vi "Switch Counter Signal.vi"(4 "Valid Signal Name":string, 5 "Counter Valid GUID":string, 6 "Counter Valid Name":string, 7 "Incoming Frame GUID":string, 8 "error in (no error)":errorcluster, 9 "Signal Page GUID":string, 10 "Counter Value GUID":string, 11 "Node Ptr":T1 format="%.0x") -> (0 "error out":errorcluster)   [LabVIEW 2015, in "Protection and Counter Support System Explorer.lvlib"]
uses:
  Protection and Counter Support System Explorer.lvlib
  <vilib>/NI Veristand/Custom Device API/Custom Device Item Ref.ctl
  <vilib>/NI Veristand/Custom Device API/Custom Device Channel Type.ctl
  <vilib>/NI Veristand/Custom Device API/Custom Device Channel.ctl
  Shared/Properties Lookup.vi
  <vilib>/NI Veristand/Custom Device API/Set Item Property (String).vi
  <vilib>/NI VeriStand/Custom Device API/Custom Device API.lvlib
  <vilib>/NI VeriStand/Custom Device Tools/Custom Device Utility Library/Custom Device Utility Library.lvlib
  Shared/Protection and Counter Support Shared.lvlib
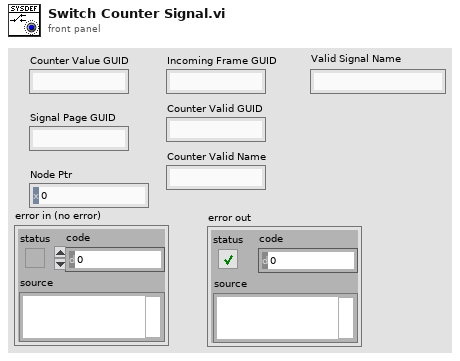
[diagram p1: front panel]
types:
  T1 = typedef "Custom Device API.lvlib/Custom Device Item Ref.ctl" = u64
  T2 = typedef "Custom Device API.lvlib/Custom Device Channel Type.ctl" = enum16{"Input", "Output"}
  T3 = typedef "Custom Device API.lvlib/Custom Device Channel.ctl" = cluster{"Type":T2, "Units":string, "Default Value":dbl, "Faultable":bool, "Scalable":bool}
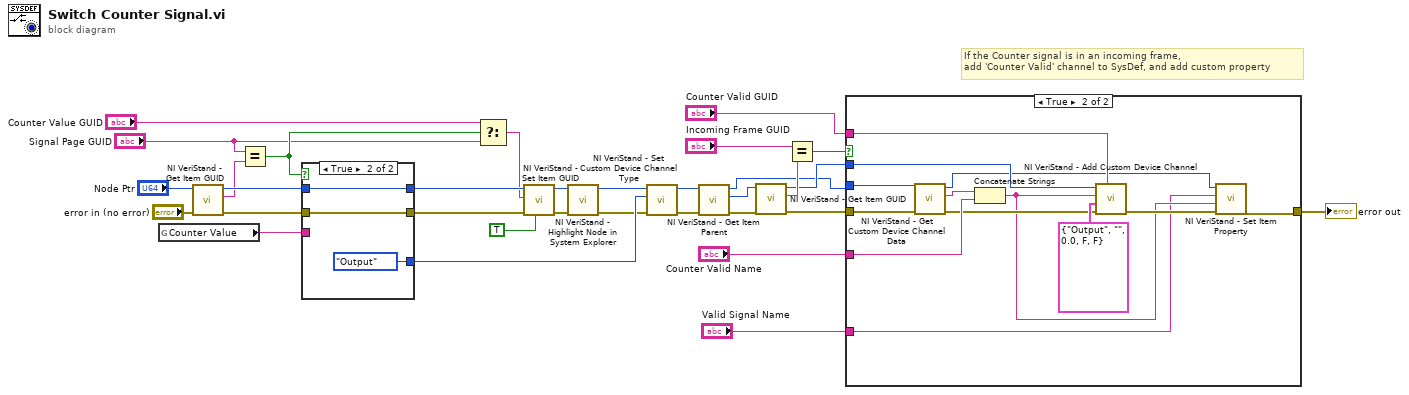
[diagram p0: block diagram]
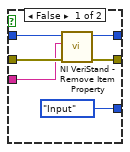
[diagram p3: hidden frame]
diagram:
  # "If the Counter signal is in an incoming frame,\nadd 'Counter Valid' channel to SysDef, and add custom property"
  n1 = global read "Properties Lookup.vi" "Counter Value"() -> (w29:string)
  n2 = call <vilib>:"NI VeriStand - Get Item GUID.vi"("error in (no error)"="error in (no error)", "Item Ref in"="Node Ptr") -> ("error out"=w24:errorcluster, "GUID"=w17:string, "Item Ref out"=w26:T1)  [unwired: 7 in]
  n3 = Equal?(x="Signal Page GUID", y=w17) -> (x = y?=w28:bool)
  n4 = case shown="True" w28 {
    tunnel: w24 -> [w38 w40]
    tunnel: [w37 w40] -> w25
    tunnel: w26 -> [w36 w41]
    tunnel: [w35 w41] -> w27
    tunnel: w29 -> [w34 _]
    tunnel: [Custom_Device_Channel_Type."Input" ("Type") Custom_Device_Channel_Type."Output" ("Type")] -> w32
    frame False {
      n5 = call <vilib>:"NI VeriStand - Remove Item Property.vi"("error in (no error)"=w38, "Property Name"=w34, "Item Ref in"=w36) -> ("error out"=w37:errorcluster, "Item Ref out"=w35:T1)  [unwired: 6 in, 1 out]
    }
    frame True {
    }
  }
  n6 = Select(t="Counter Value GUID", s=w28, f="Signal Page GUID") -> (s? t:f=w19:string)
  n7 = call <vilib>:"NI VeriStand - Set Item GUID.vi"("Refresh System Explorer Tree? (F)"=TRUE, "error in (no error)"=w25, "GUID"=w19, "Item Ref in"=w27) -> ("error out"=w22:errorcluster, "Item Ref out"=w23:T1)  [unwired: 6 in]
  n8 = call <vilib>:"NI VeriStand - Highlight Node in System Explorer.vi"("error in (no error)"=w22, "Item Ref in"=w23) -> ("error out"=w30:errorcluster, "Node Ptr dup"=w31:T1)  [unwired: 8 in]
  n9 = call <vilib>:"NI VeriStand - Set Custom Device Channel Type.vi"("error in (no error)"=w30, "Type"=w32, "Channel Ref in"=w31) -> ("error out"=w14:errorcluster, "Channel Ref out"=w13:T1)  [unwired: 7 in]
  n10 = call <vilib>:"NI VeriStand - Get Item Parent.vi"("error in (no error)"=w14, "Item Ref in"=w13) -> ("error out"=w12:errorcluster, "Parent Ref"=w4:T1, "Item Ref out"=w2:T1)  [unwired: 6 in, 1 out]
  n11 = call <vilib>:"NI VeriStand - Get Item GUID.vi"("error in (no error)"=w12, "Item Ref in"=w4) -> ("error out"=w11:errorcluster, "GUID"=w9:string, "Item Ref out"=w3:T1)  [unwired: 7 in]
  n12 = Equal?(x="Incoming Frame GUID", y=w9) -> (x = y?=w7:bool)
  n13 = case shown="True" w7 {
    tunnel: w11 -> [w42 w49]
    tunnel: w3 -> [_ w55]
    tunnel: [w42 w43] -> w10
    tunnel: "Counter Valid GUID" -> [_ w54]
    tunnel: "Counter Valid Name" -> [_ w50]
    tunnel: w2 -> [_ w52]
    tunnel: "Valid Signal Name" -> [_ w44]
    frame False {
    }
    frame True {
      n14 = call <vilib>:"NI VeriStand - Get Custom Device Channel Data.vi"("error in (no error)"=w49, "Channel Ref in"=w52) -> ("error out"=w48:errorcluster, "Channel Name"=w51:string, "Channel Ref out"=w46:T1)  [unwired: 4 in, 3 out]
      n15 = Concatenate Strings(w51, w50) -> (w45:string)
      n16 = call <vilib>:"NI VeriStand - Add Custom Device Channel.vi"("GUID (Default Channel)"=w54, "error in (no error)"=w48, "Channel"=T3 {"Type"=enum."Output", "Units"="", "Default Value"=0.0, "Faultable"=FALSE, "Scalable"=FALSE}, "Channel Name"=w45, "Parent Ref in"=w55) -> ("error out"=w47:errorcluster)  [unwired: 3 in, 3 out]
      n17 = call-poly <vilib>:"NI VeriStand - Set Item Property.vi"("error in (no error)"=w47, "Value"=w45, "Property Name"=w44, "Item Ref in"=w46) -> ("error out"=w43:errorcluster)  [unwired: 5 in, 2 out]
    }
  }
  "error out" <- w10
